vi "读取数据解析(子VI).vi"(6 "数据":string, 7 "命令编码CN":string, 11 "队列输入":refnum<queue>) -> (0 "实时数据发送时间间隔/min":i32=1, 1 "元素":T1(ring), 2 "设置超时时间/min":i32=1, 3 "队列输出":refnum<queue>, 4 "table":string="提取监测仪表时间")   [LabVIEW 2016, in "数据传输系统.lvlib"]
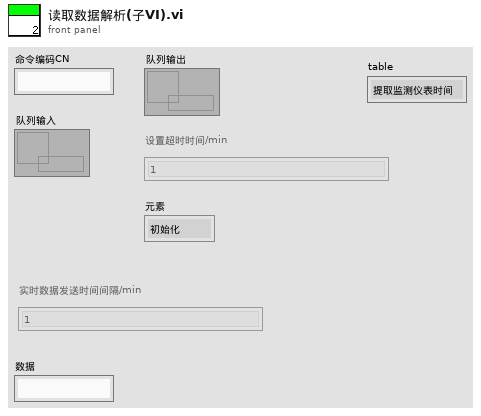
[diagram p1: front panel]
types:
  T1 = enum16{"初始化", "打开连接", "表格比对", "发送数据", "读取数据", "数据处理"}
  T2 = enum16{"CODMn", "CODCr", "氨氮", "总磷", "总氮", "数采仪"}
  T3 = cluster{"高锰酸盐":string, "化学需氧量":string, "氨氮":string, "总磷":string, "总氮":string, "数采仪":string, "高锰酸盐":bool, "化学需氧量":bool, "氨氮":bool, "总磷":bool, "总氮":bool, "数采仪":bool}
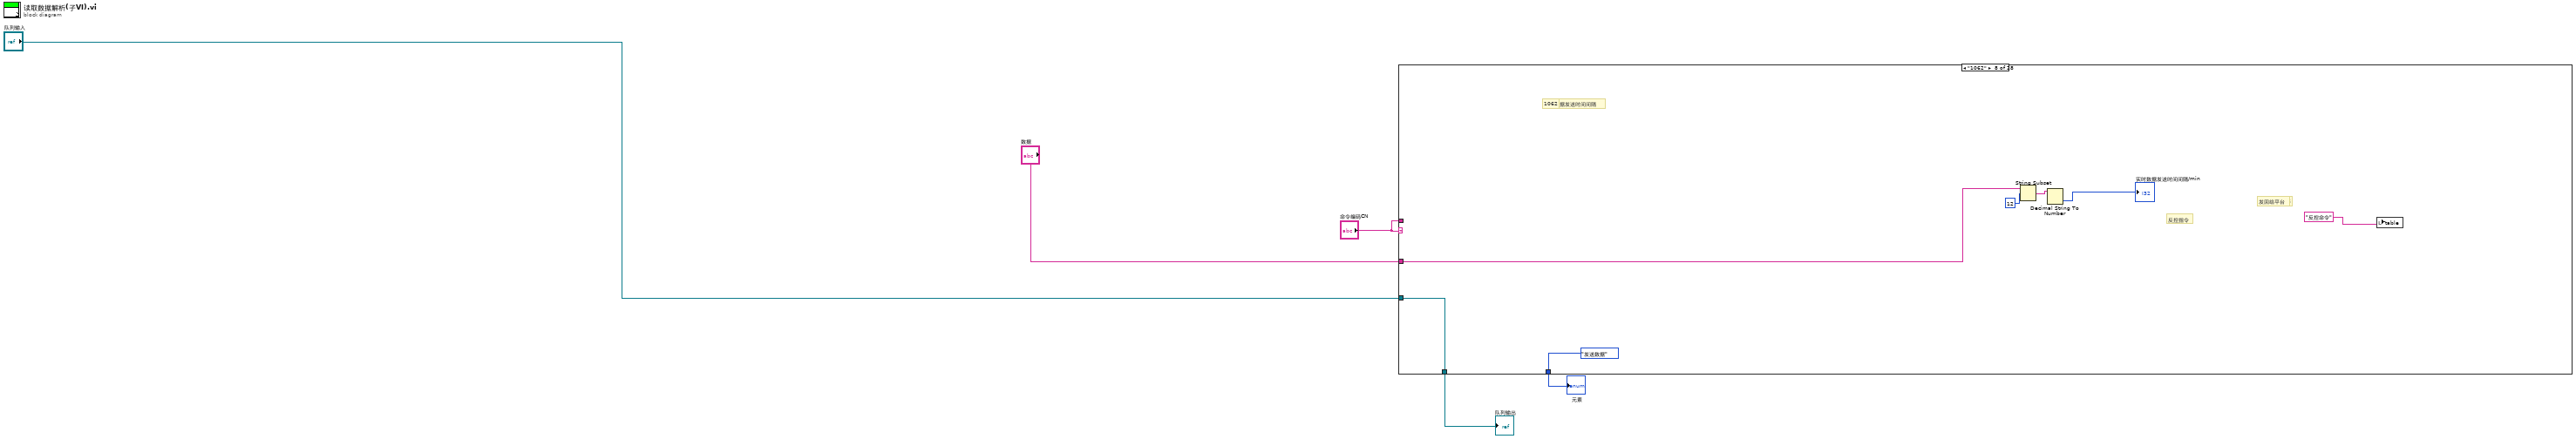
[diagram p0: block diagram]
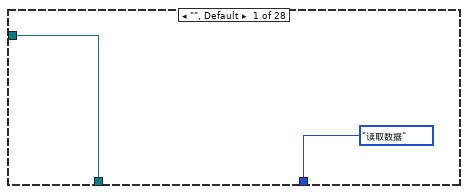
[diagram p2: hidden frame]
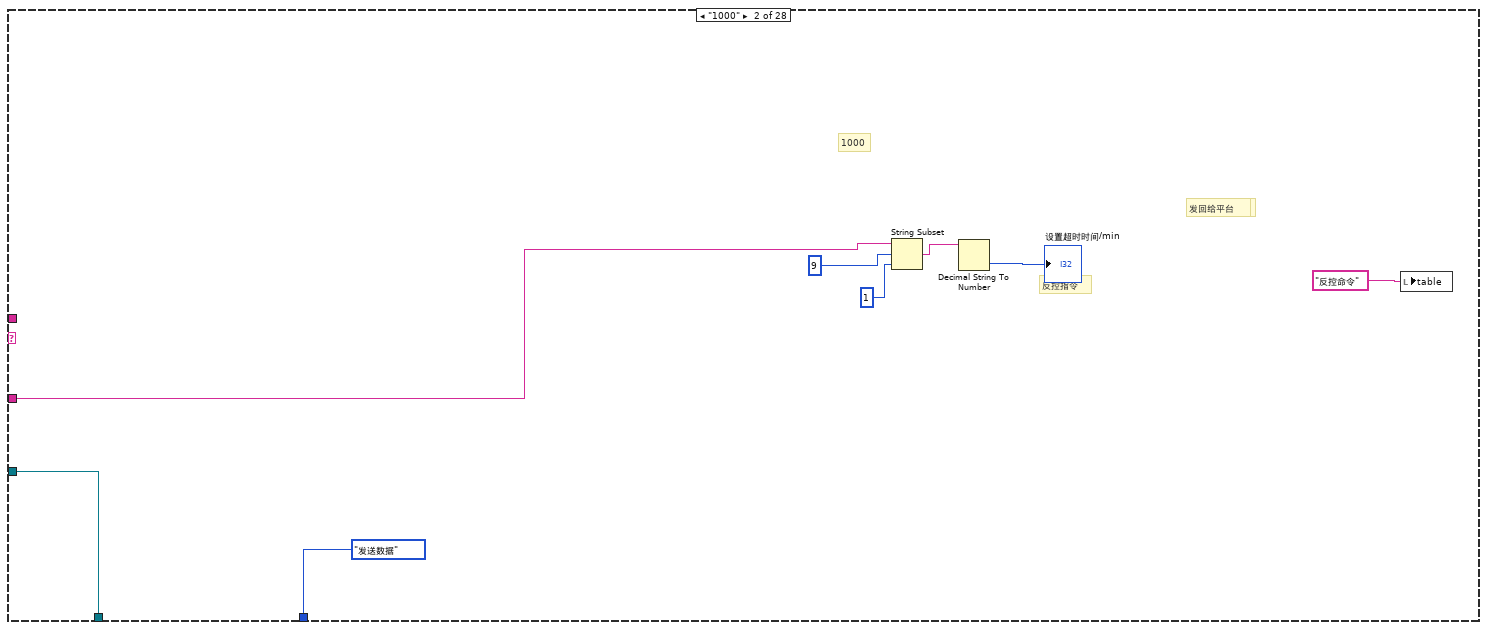
[diagram p3: hidden frame]
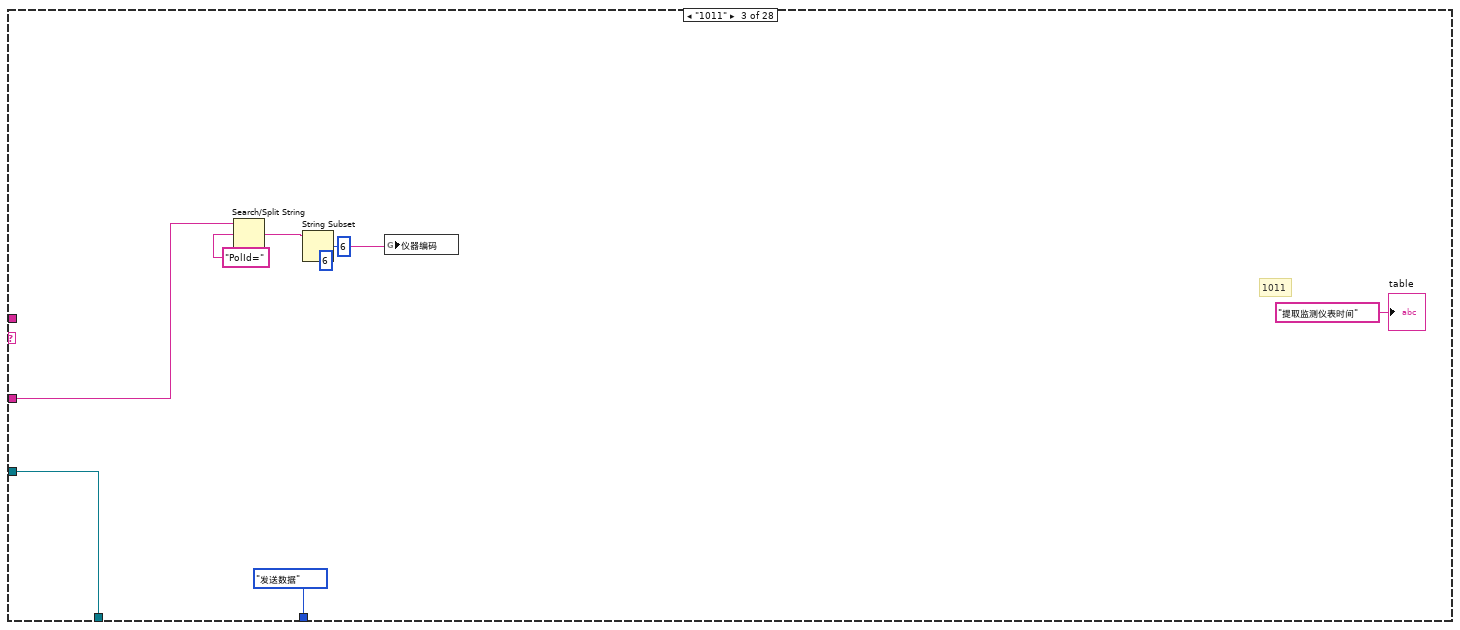
[diagram p4: hidden frame]
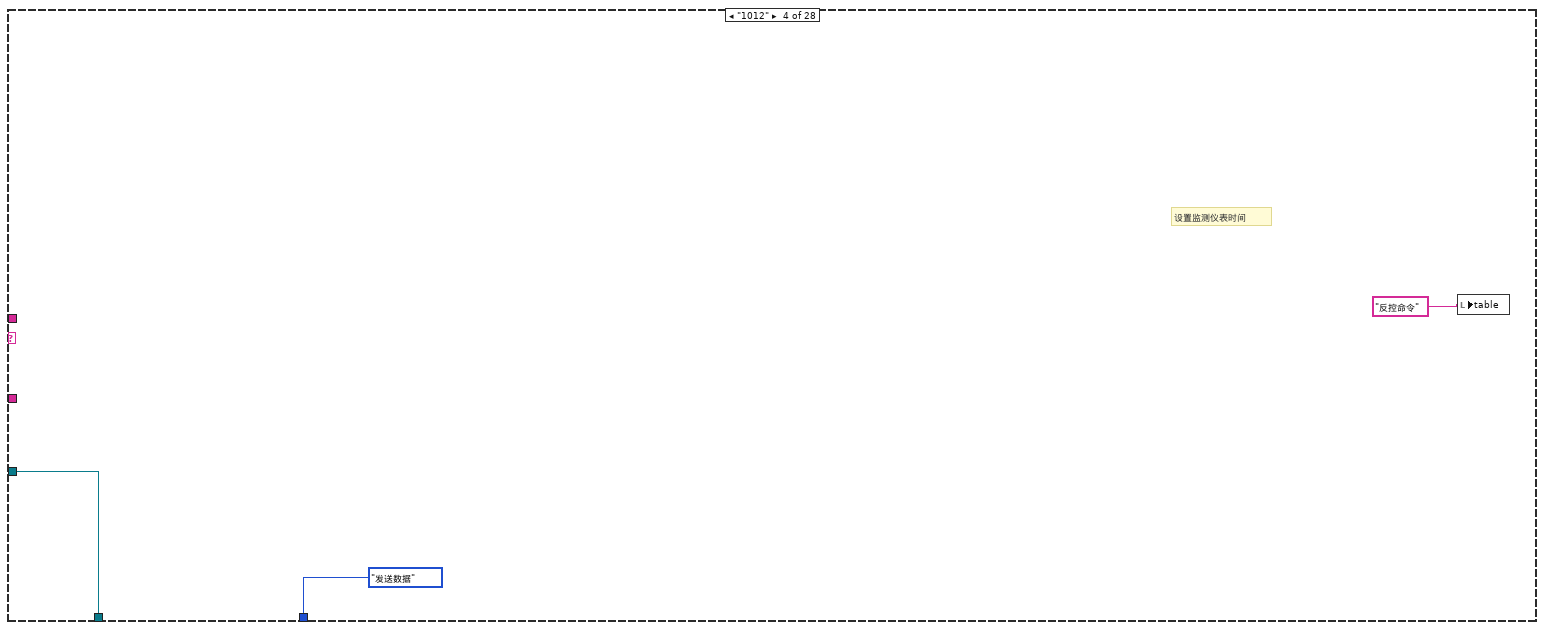
[diagram p5: hidden frame]
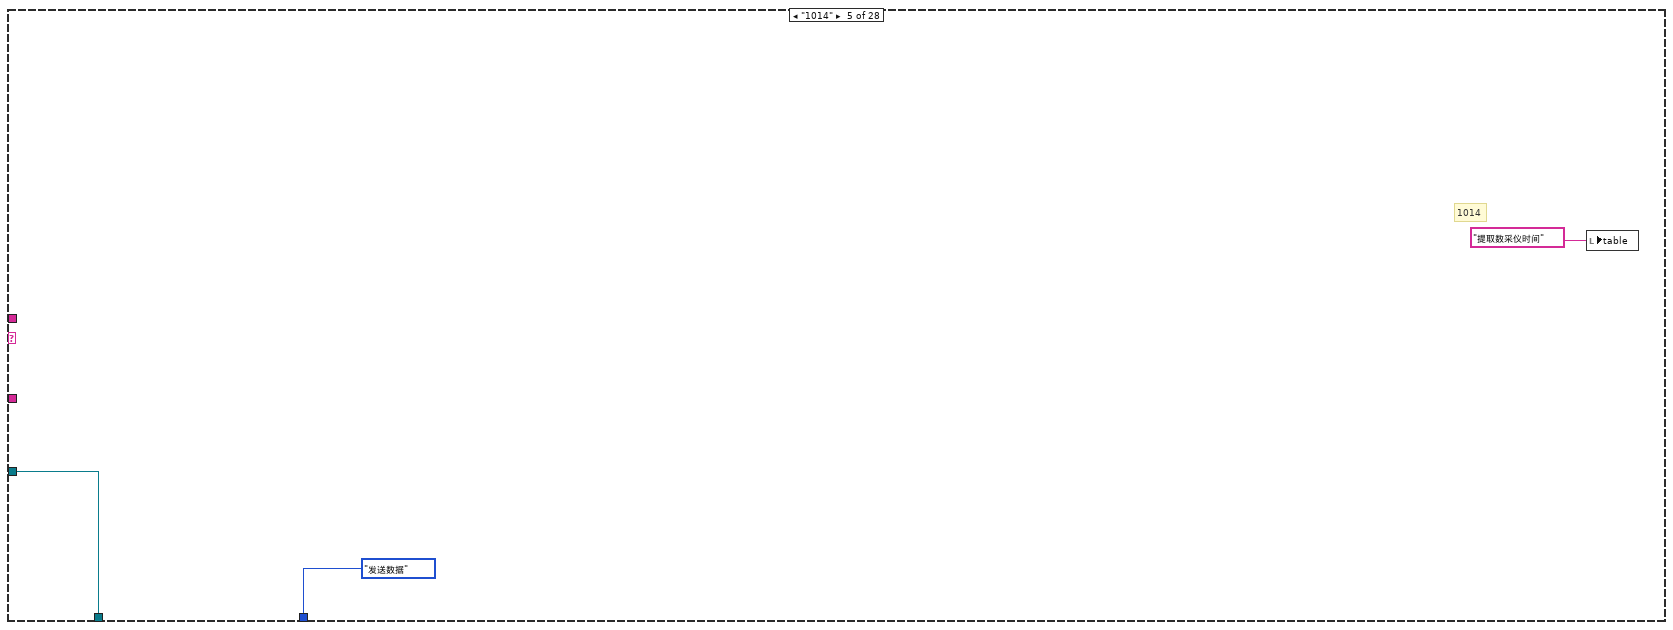
[diagram p6: hidden frame]
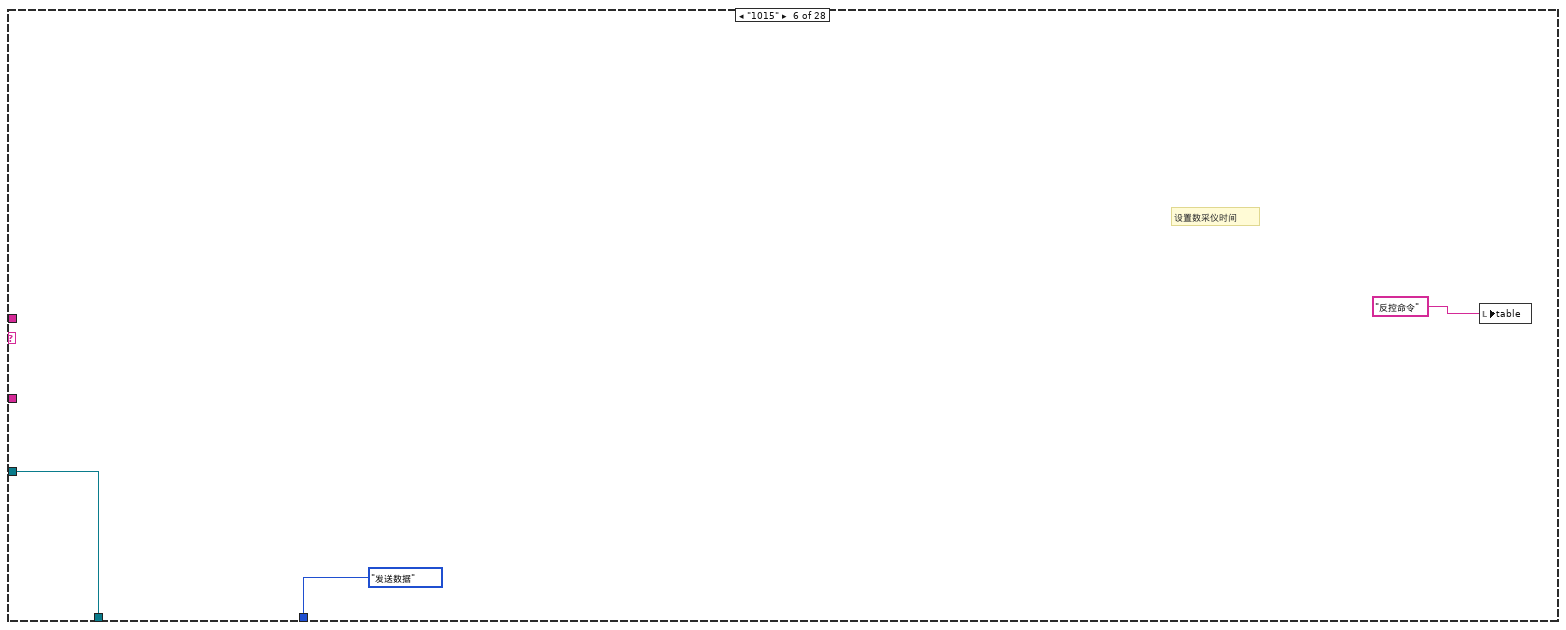
[diagram p7: hidden frame]
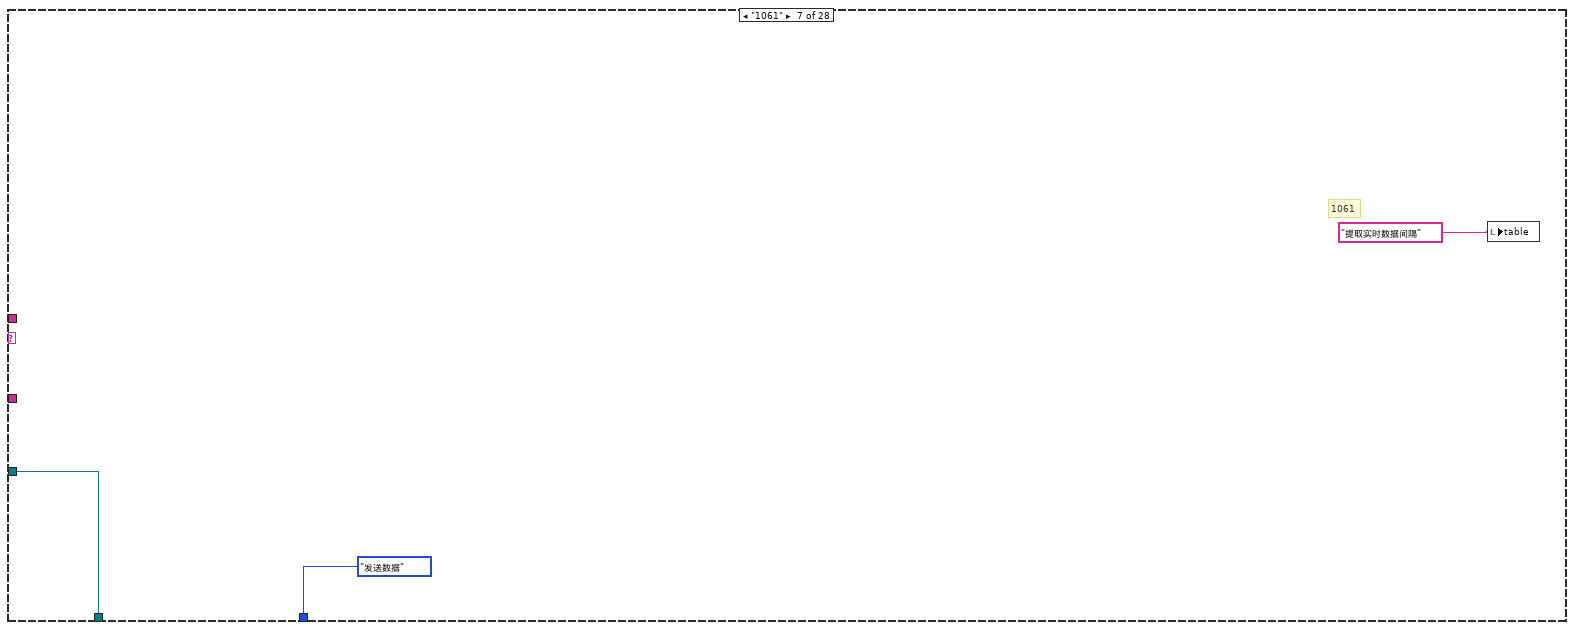
[diagram p8: hidden frame]
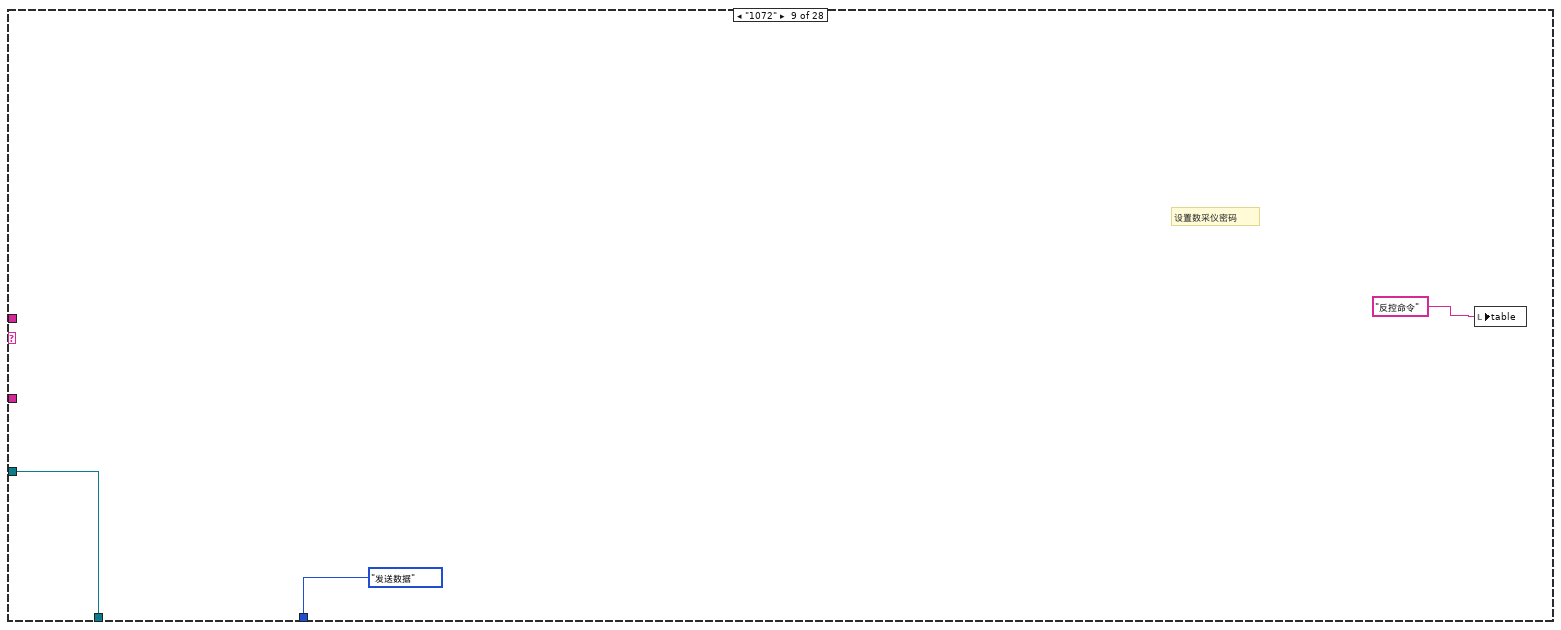
[diagram p9: hidden frame]
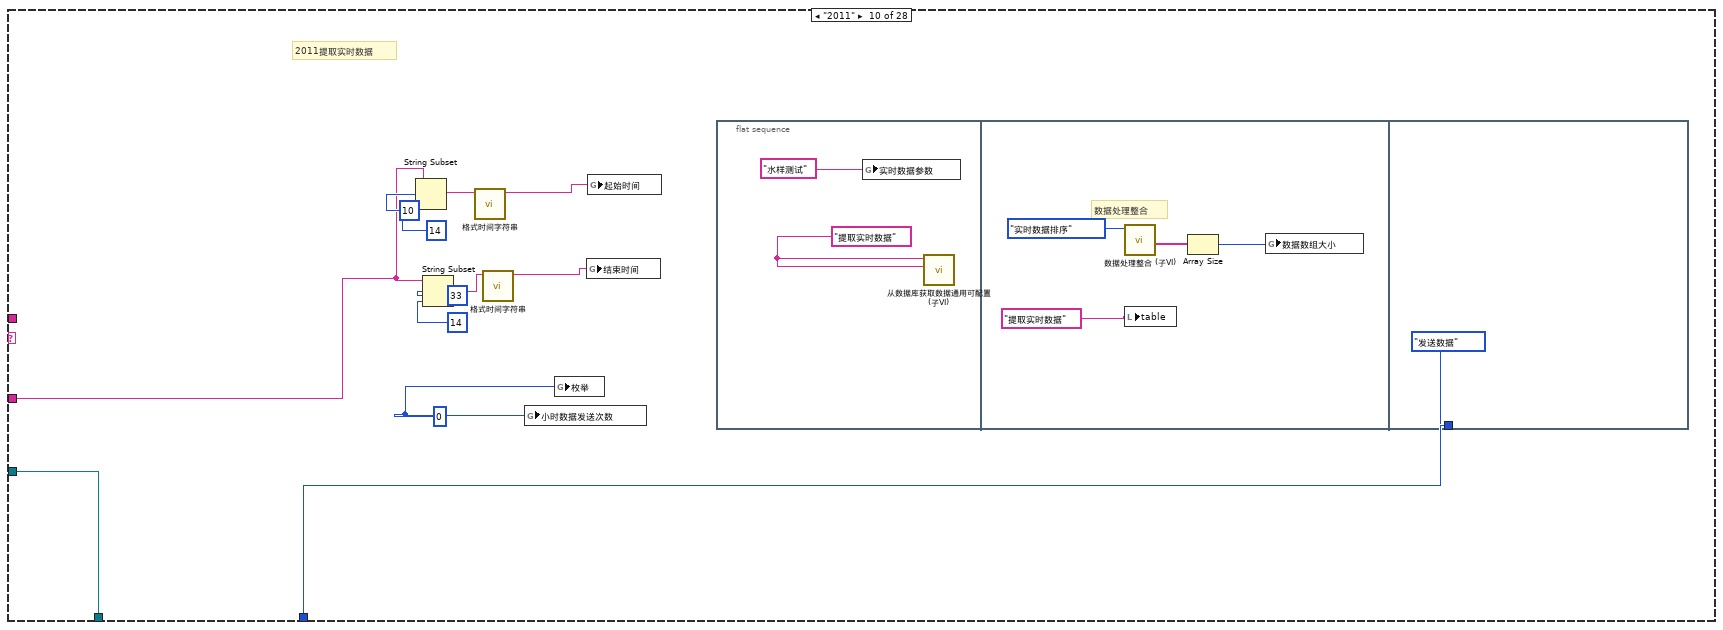
[diagram p10: hidden frame]
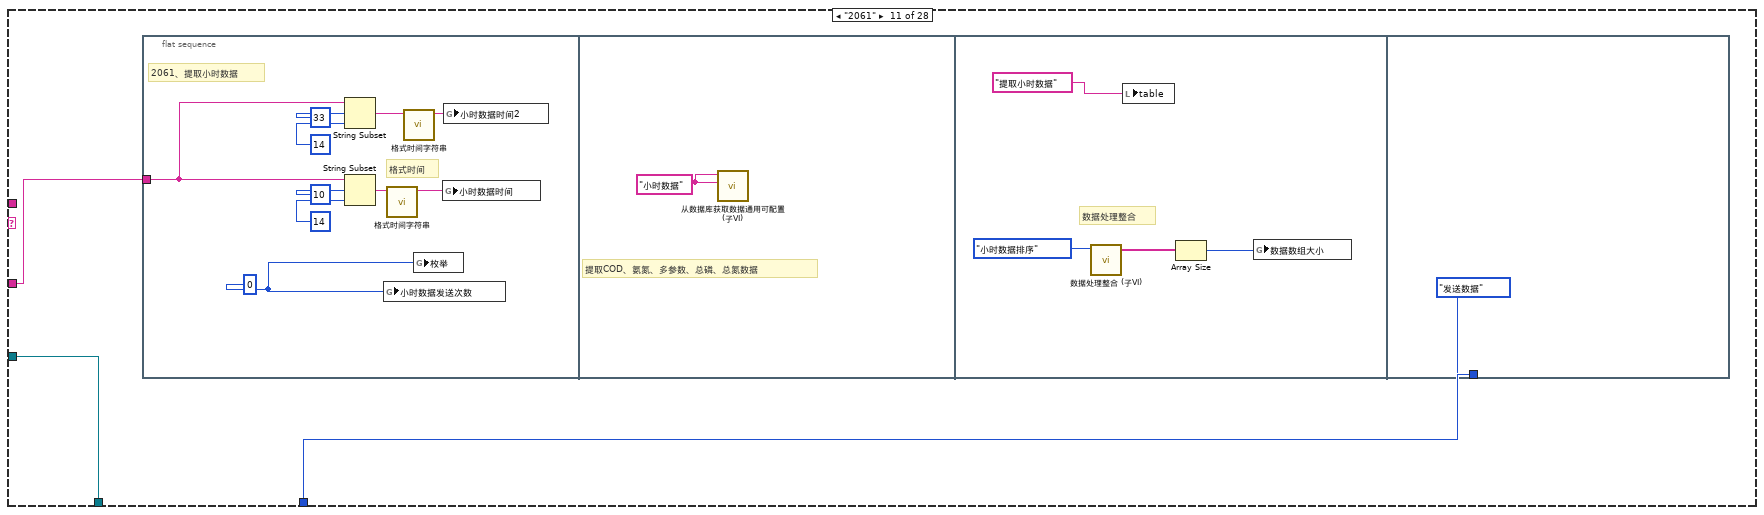
[diagram p11: hidden frame]
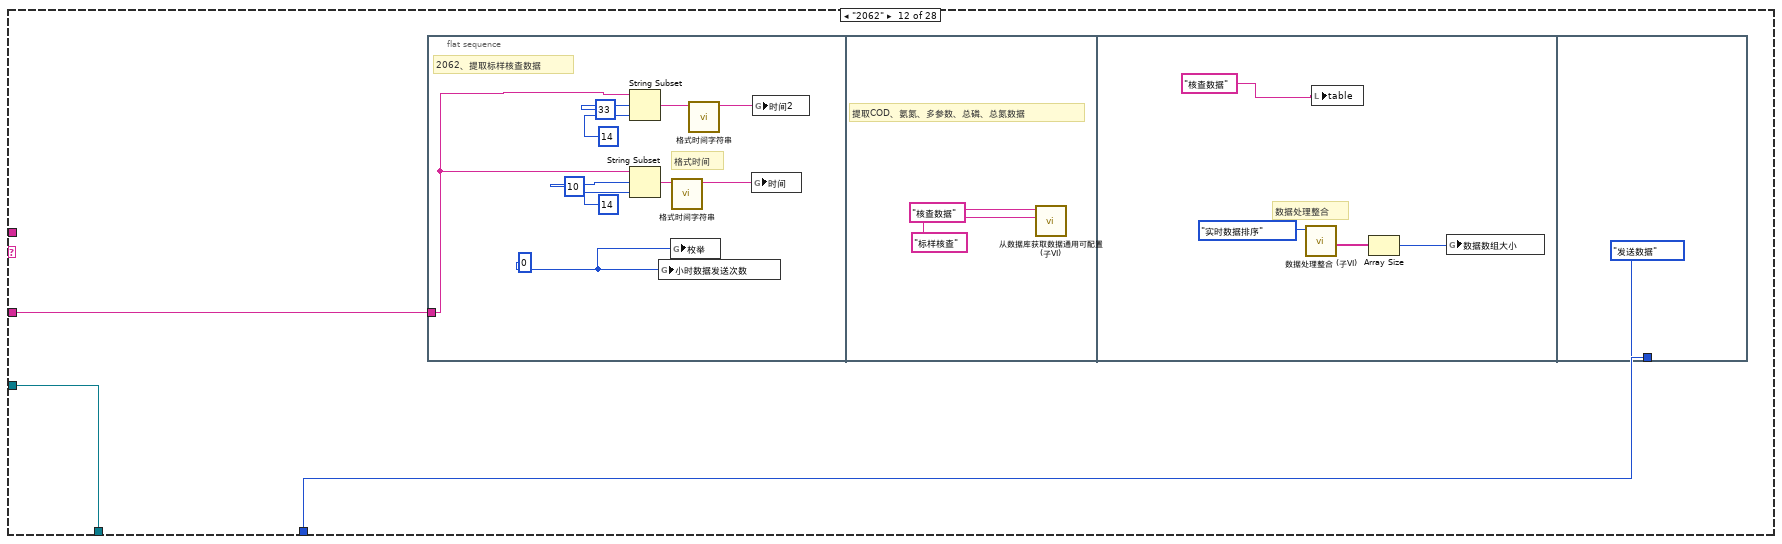
[diagram p12: hidden frame]
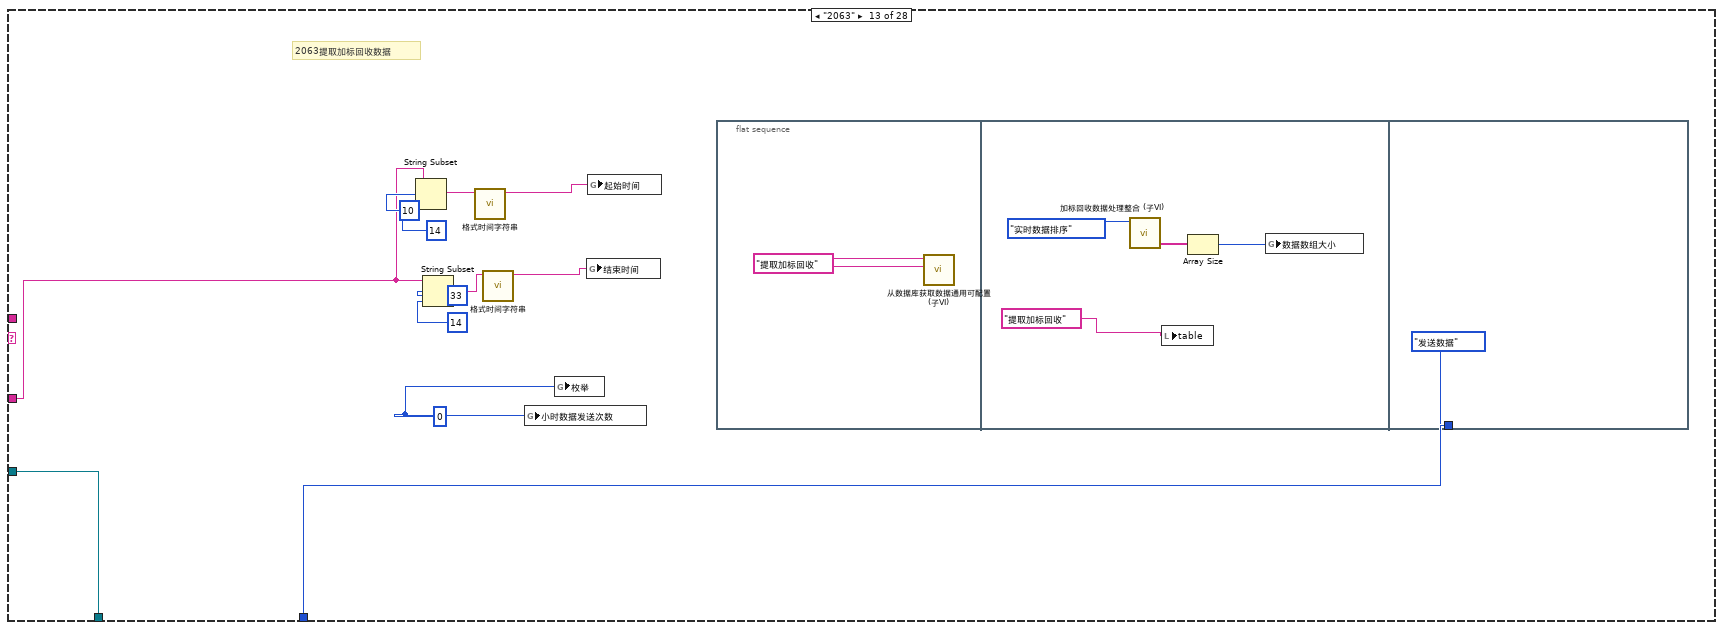
[diagram p13: hidden frame]
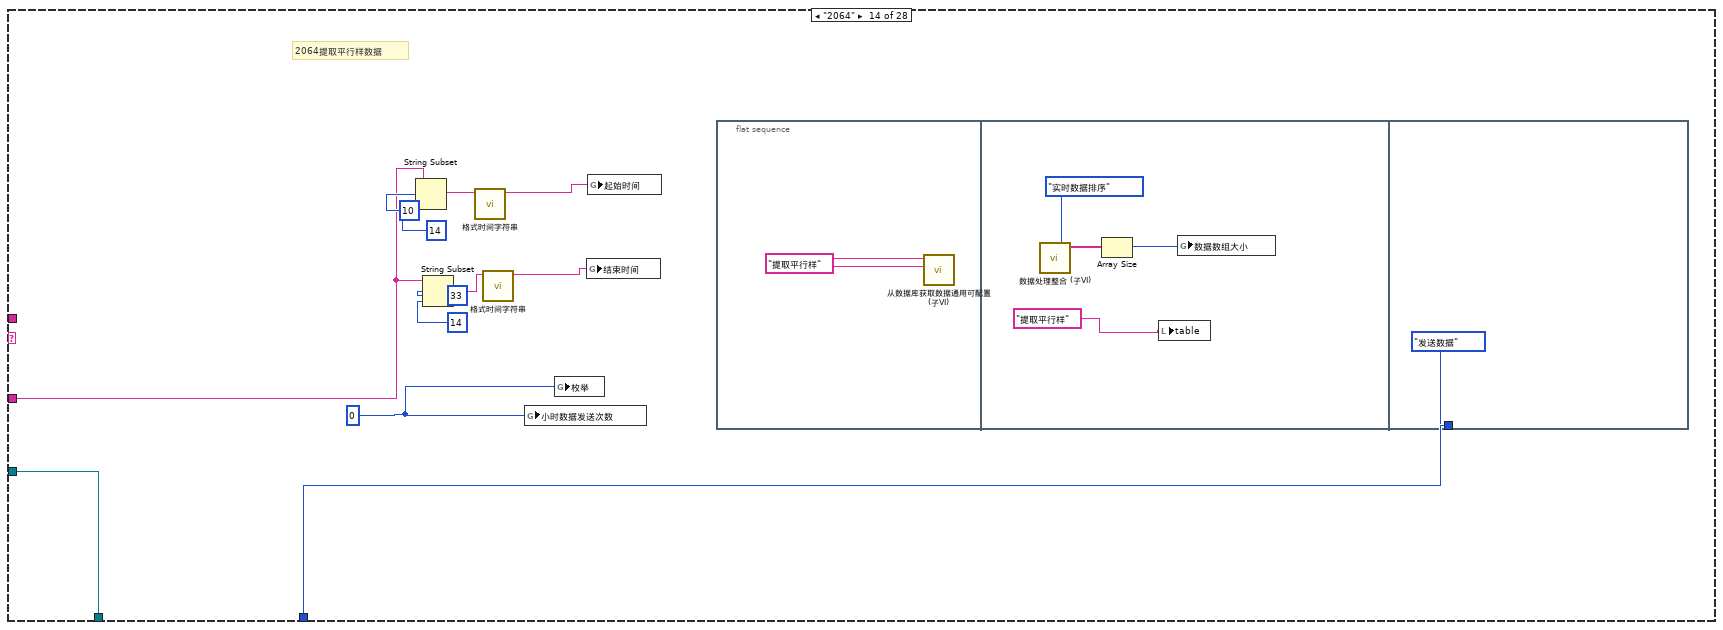
[diagram p14: hidden frame]
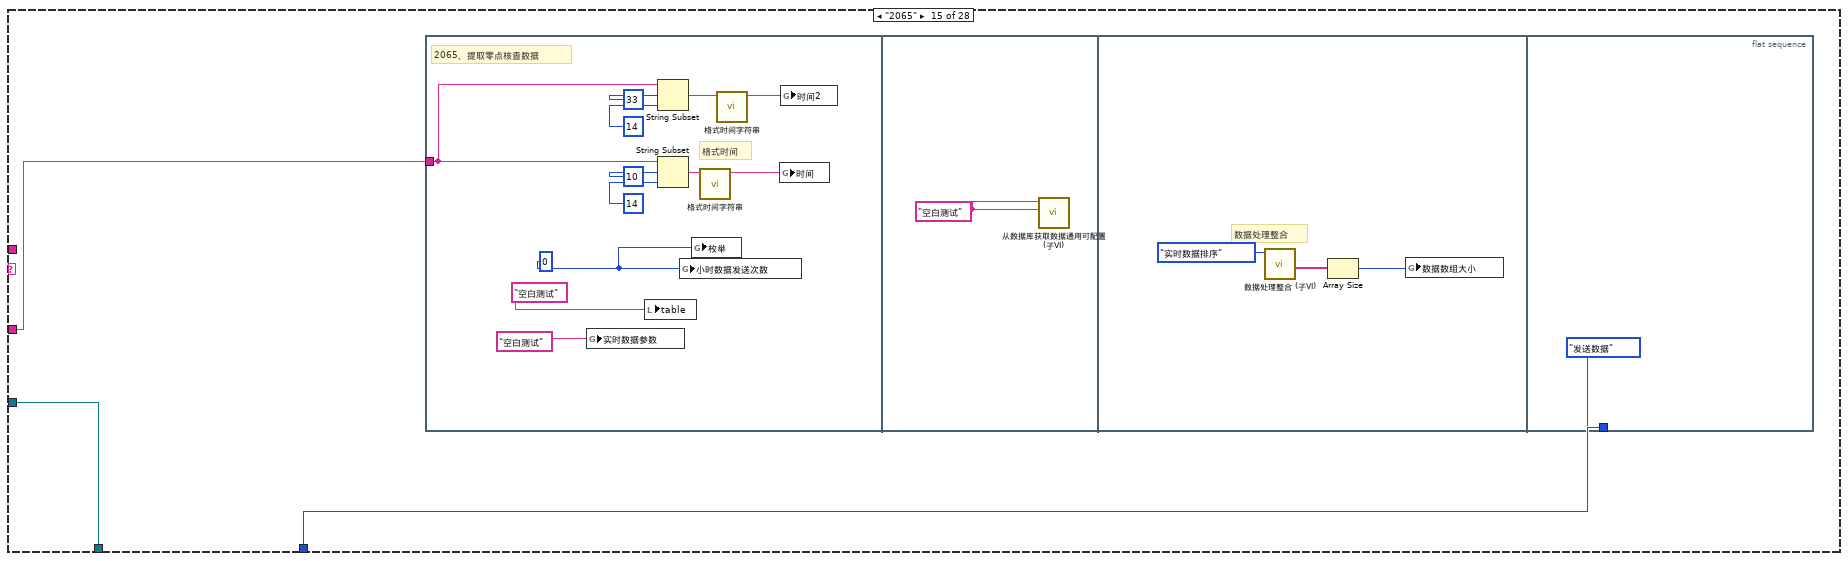
[diagram p15: hidden frame]
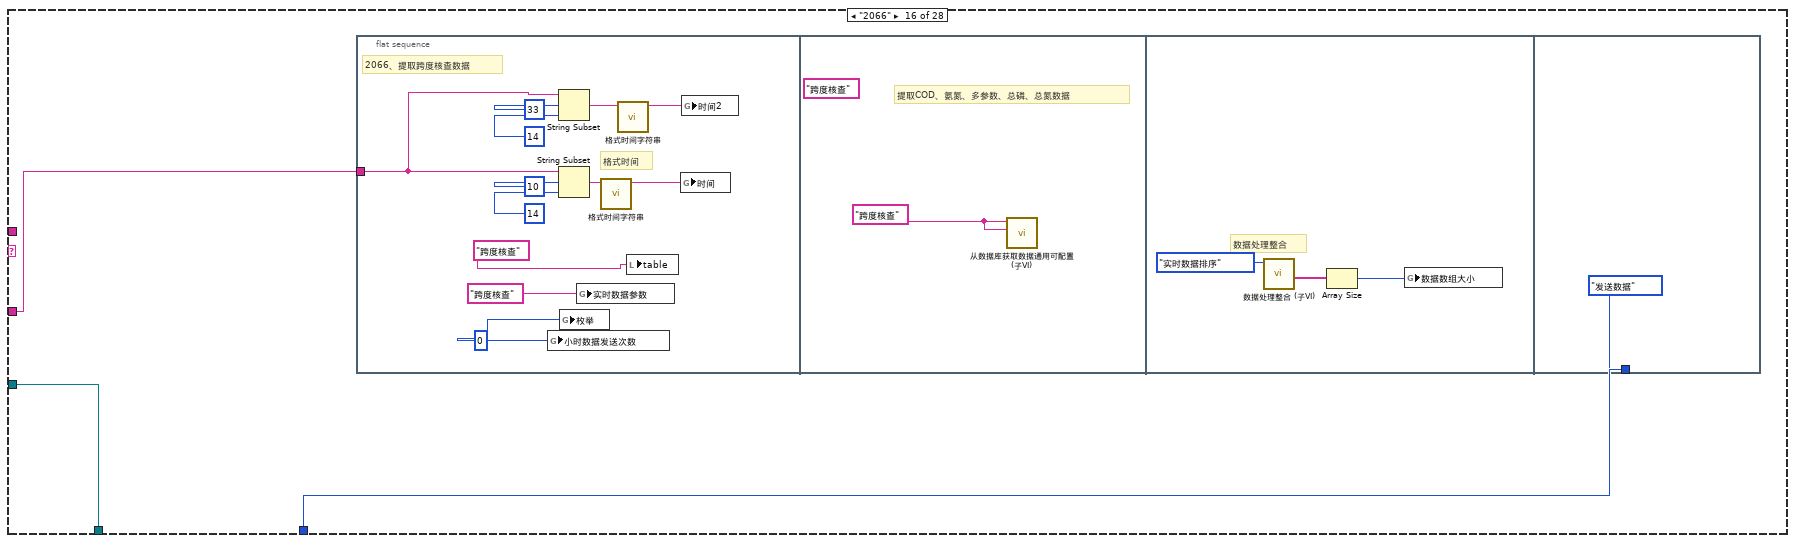
[diagram p16: hidden frame]
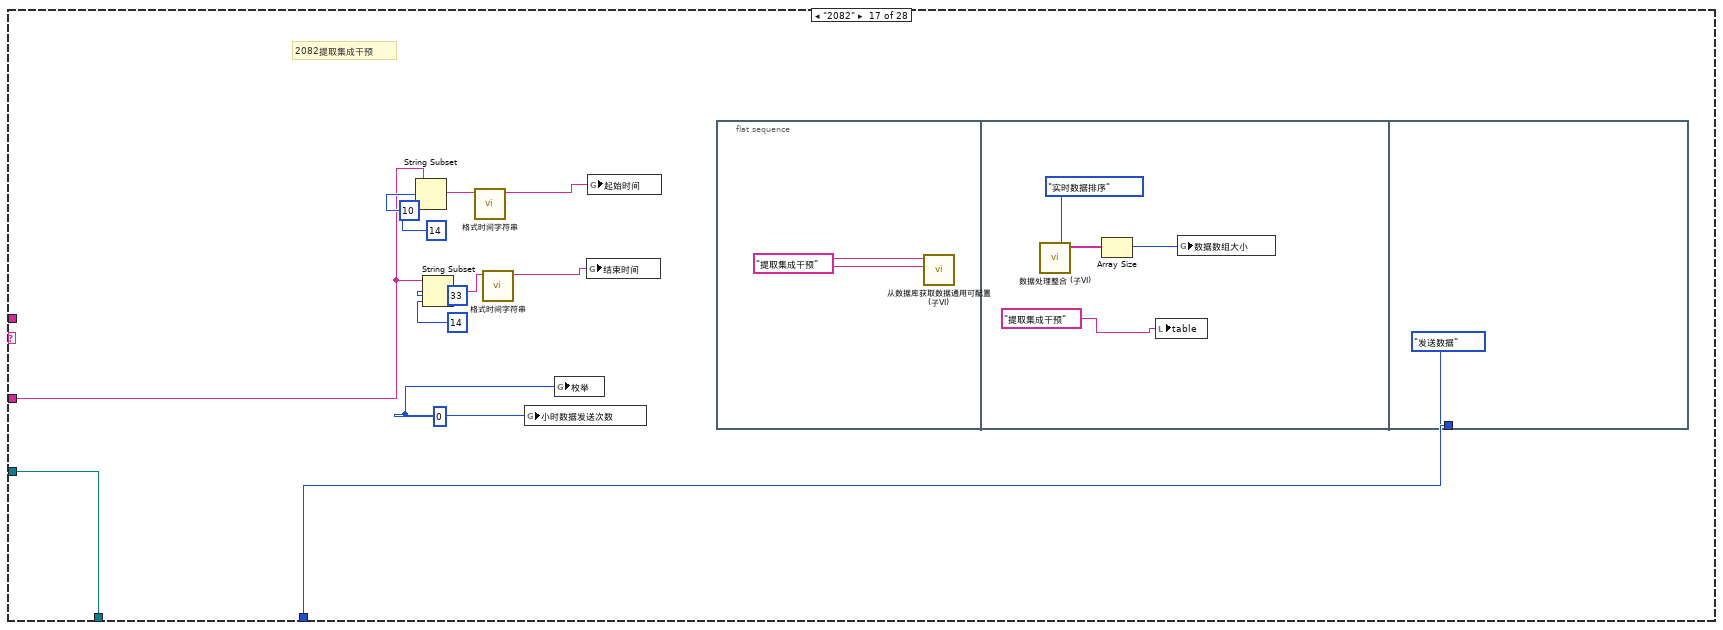
[diagram p17: hidden frame]
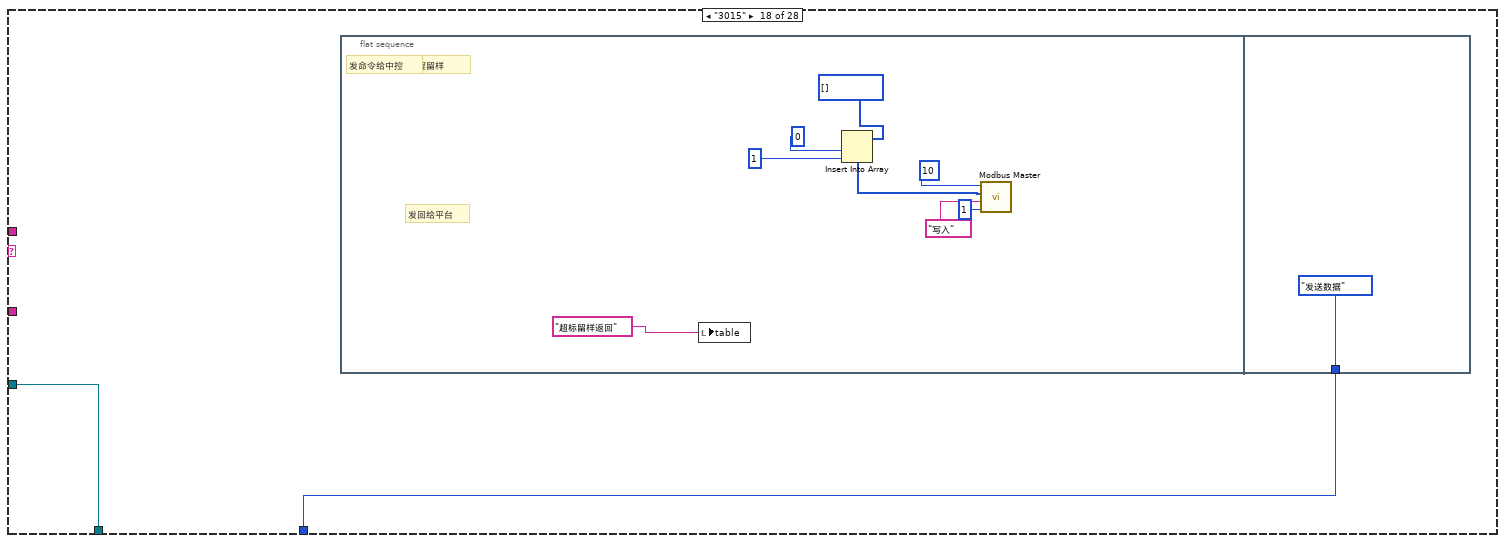
[diagram p18: hidden frame]
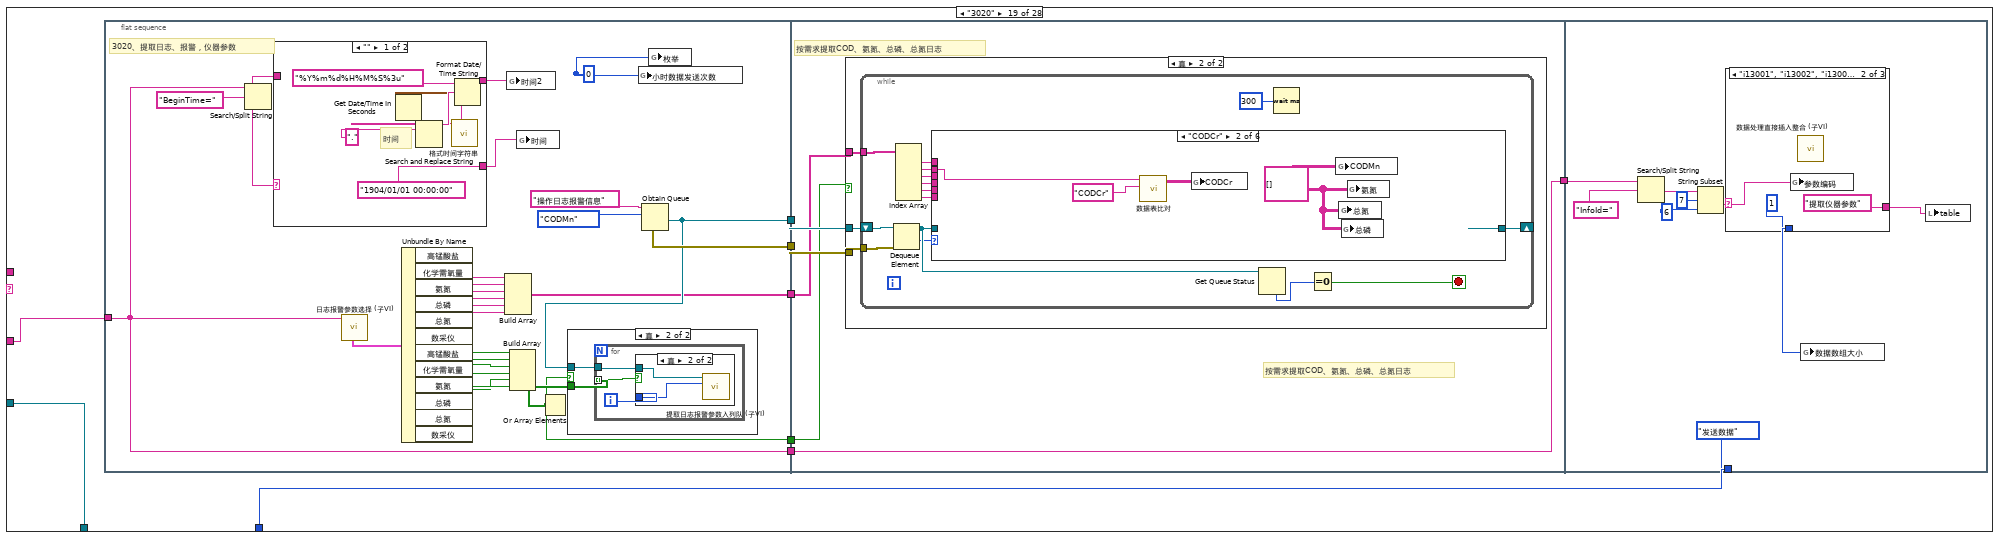
[diagram p19: hidden frame]
diagram:
  n1 = case shown="\"1062\"" "命令编码CN" {
    tunnel: "队列输入" -> [w7 w11 w24 w27 w30 w33 w36 w41 w46 w49 w68 w87 w107 w125 w143 w163 w183 w200 w218 w341 w343 w347 w355 w372 w375 w387 w409 w416]
    tunnel: [w7 w11 w24 w27 w30 w33 w36 w41 w46 w49 w68 w87 w107 w125 w143 w163 w183 w200 w218 w341 w343 w347 w355 w372 w375 w387 w409 w416] -> w2
    tunnel: [T1."读取数据" ("元素") T1."发送数据" ("元素") T1."发送数据" ("元素") T1."发送数据" ("元素") T1."发送数据" ("元素") T1."发送数据" ("元素") T1."发送数据" ("元素") T1."发送数据" ("元素") T1."发送数据" ("元素") w48 w67 w86 w106 w124 w142 w162 w182 w199 w217 T1."发送数据" ("元素") w342 w346 T1."发送数据" ("元素") T1."发送数据" ("元素") T1."发送数据" ("元素") T1."发送数据" ("元素") T1."发送数据" ("元素") T1."发送数据" ("元素")] -> w3
    tunnel: "命令编码CN" -> [_ _ _ _ _ _ _ _ _ _ _ _ _ _ _ _ _ _ _ _ _ _ _ _ _ _ _ w415]
    tunnel: "数据" -> [_ w9 w17 _ _ _ _ w39 _ w47 w66 w85 w105 w123 w141 w161 w181 _ w212 _ _ _ w351 _ _ _ w398 w412]
    frame "", Default {
    }
    frame "1000" {
      # "发回给平台"
      # "反控指令"
      # "3042~3086"
      # "1000"
      n2 = String Subset(string=w9, offset (0)=9 ("偏移量(0)"), length (rest)=1 ("长度（剩余）")) -> (substring=w13:string)
      n3 = Decimal String To Number(string=w13) -> (number=→"设置超时时间/min":i32)  [unwired: 2 in, 1 out]
      n4 = local write "table"("反控命令" ("新元素/子数组")) -> ()
    }
    frame "1011" {
      # "1011"
      n5 = Search/Split String(string=w17, search string/char (-)="PolId=" ("搜索字符串/字符(-)")) -> (match + rest of string=w21:string)  [unwired: 1 in, 2 out]
      n6 = String Subset(string=w21, offset (0)=6 ("偏移量(0)"), length (rest)=6 ("长度（剩余）")) -> (substring=w18:string)
      n7 = global write "全局 提取仪器参数.vi" "仪器编码"(w18) -> ()
      "table" <- "提取监测仪表时间"
    }
    frame "1012" {
      # "设置监测仪表时间"
      n8 = local write "table"("反控命令" ("新元素/子数组")) -> ()
    }
    frame "1014" {
      # "1014"
      n9 = local write "table"("提取数采仪时间") -> ()
    }
    frame "1015" {
      # "设置数采仪时间"
      n10 = local write "table"("反控命令" ("新元素/子数组")) -> ()
    }
    frame "1061" {
      # "1061"
      n11 = local write "table"("提取实时数据间隔") -> ()
    }
    frame "1062" {
      # "发回给平台"
      # "反控指令"
      # "3042~3086"
      # "设置数据发送时间间隔"
      # "1062"
      n12 = String Subset(string=w39, offset (0)=12 ("偏移量(0)")) -> (substring=w42:string)  [unwired: 1 in]
      n13 = Decimal String To Number(string=w42) -> (number=→"实时数据发送时间间隔/min":i32)  [unwired: 2 in, 1 out]
      n14 = local write "table"("反控命令" ("新元素/子数组")) -> ()
    }
    frame "1072" {
      # "设置数采仪密码"
      n15 = local write "table"("反控命令" ("新元素/子数组")) -> ()
    }
    frame "2011" {
      w54 = 0 ("数值")
      # "2011提取实时数据"
      n16 = String Subset(string=w47, offset (0)=10 ("偏移量(0)"), length (rest)=14 ("长度（剩余）")) -> (substring=w51:string)
      n17 = String Subset(string=w47, offset (0)=33 ("偏移量(0)"), length (rest)=14 ("长度（剩余）")) -> (substring=w53:string)
      n18 = call "格式时间字符串.vi"("字符串"=w51) -> ("连接的字符串"=w50:string)  [unwired: 10 in]
      n19 = call "格式时间字符串.vi"("字符串"=w53) -> ("连接的字符串"=w52:string)  [unwired: 10 in]
      n20 = global write "全局 小时数据发送次数.vi" "小时数据发送次数"(w54) -> ()
      n21 = global write "全局1.vi" "枚举"(w54) -> ()
      n22 = global write "起始时间.vi" "结束时间"(w52) -> ()
      n23 = global write "起始时间.vi" "起始时间"(w50) -> ()
      n24 = flat-sequence {
        tunnel: [T1."发送数据" ("元素")] -> w48
        frame #0 {
          w59 = "提取实时数据" ("新元素/子数组")
          n25 = global write "全局 实时数据参数.vi" "实时数据参数"("水样测试") -> ()
          n26 = call "从数据库获取数据通用可配置(子VI).vi"("table输入"=w59, "列队名（唯一）"=w59) -> ()  [unwired: 8 in, 2 out]
        }
        frame #1 {
          # "数据处理整合"
          n27 = call "数据处理整合 (子VI).vi"("枚举"=enum16{"实时数据排序", "小时数据排序"}."实时数据排序") -> ("已排序的数组"=w63:string[])  [unwired: 10 in]
          n28 = local write "table"("提取实时数据" ("新元素/子数组")) -> ()
          n29 = Array Size(array=w63) -> (size(s)=w64:i32)
          n30 = global write "全局 数据数组大小.vi" "数据数组大小"(w64) -> ()
        }
        frame #2 {
        }
      }
    }
    frame "2061" {
      n31 = flat-sequence {
        tunnel: w66 -> [w69]
        tunnel: [T1."发送数据" ("元素")] -> w67
        frame #0 {
          w70 = 0 ("数值")
          # "格式时间"
          # "2061、提取小时数据"
          n32 = String Subset(string=w69, offset (0)=33 ("偏移量(0)"), length (rest)=14 ("长度（剩余）")) -> (substring=w72:string)
          n33 = String Subset(string=w69, offset (0)=10 ("偏移量(0)"), length (rest)=14 ("长度（剩余）")) -> (substring=w73:string)
          n34 = global write "全局 小时数据发送次数.vi" "小时数据发送次数"(w70) -> ()
          n35 = call "格式时间字符串.vi"("字符串"=w73) -> ("连接的字符串"=w74:string)  [unwired: 10 in]
          n36 = call "格式时间字符串.vi"("字符串"=w72) -> ("连接的字符串"=w71:string)  [unwired: 10 in]
          n37 = global write "全局1.vi" "枚举"(w70) -> ()
          n38 = global write "全局 水样时间.vi" "小时数据时间"(w74) -> ()
          n39 = global write "全局 时间2.vi" "小时数据时间2"(w71) -> ()
        }
        frame #1 {
          w79 = "小时数据" ("名称（未命名）")
          # "提取COD、氨氮、多参数、总磷、总氮数据"
          n40 = call "从数据库获取数据通用可配置(子VI).vi"("table输入"=w79, "列队名（唯一）"=w79) -> ()  [unwired: 8 in, 2 out]
        }
        frame #2 {
          # "数据处理整合"
          n41 = call "数据处理整合 (子VI).vi"("枚举"=enum16{"实时数据排序", "小时数据排序"}."小时数据排序") -> ("已排序的数组"=w83:string[])  [unwired: 10 in]
          n42 = local write "table"("提取小时数据" ("新元素/子数组")) -> ()
          n43 = Array Size(array=w83) -> (size(s)=w82:i32)
          n44 = global write "全局 数据数组大小.vi" "数据数组大小"(w82) -> ()
        }
        frame #3 {
        }
      }
    }
    frame "2062" {
      n45 = flat-sequence {
        tunnel: w85 -> [w88]
        tunnel: [T1."发送数据" ("元素")] -> w86
        frame #0 {
          w89 = 0 ("数值")
          # "格式时间"
          # "2062、提取标样核查数据"
          n46 = String Subset(string=w88, offset (0)=33 ("偏移量(0)"), length (rest)=14 ("长度（剩余）")) -> (substring=w91:string)
          n47 = String Subset(string=w88, offset (0)=10 ("偏移量(0)"), length (rest)=14 ("长度（剩余）")) -> (substring=w92:string)
          n48 = global write "全局 小时数据发送次数.vi" "小时数据发送次数"(w89) -> ()
          n49 = global write "全局1.vi" "枚举"(w89) -> ()
          n50 = call "格式时间字符串.vi"("字符串"=w92) -> ("连接的字符串"=w93:string)  [unwired: 10 in]
          n51 = call "格式时间字符串.vi"("字符串"=w91) -> ("连接的字符串"=w90:string)  [unwired: 10 in]
          n52 = global write "全局 水样时间.vi" "时间"(w93) -> ()
          n53 = global write "全局 时间2.vi" "时间2"(w90) -> ()
        }
        frame #1 {
          # "提取COD、氨氮、多参数、总磷、总氮数据"
          n54 = call "从数据库获取数据通用可配置(子VI).vi"("table输入"="标样核查" ("新元素/子数组"), "列队名（唯一）"="核查数据" ("新元素/子数组")) -> ()  [unwired: 8 in, 2 out]
        }
        frame #2 {
          # "数据处理整合"
          n55 = call "数据处理整合 (子VI).vi"("枚举"=enum16{"实时数据排序", "小时数据排序"}."实时数据排序") -> ("已排序的数组"=w102:string[])  [unwired: 10 in]
          n56 = local write "table"("核查数据" ("新元素/子数组")) -> ()
          n57 = Array Size(array=w102) -> (size(s)=w103:i32)
          n58 = global write "全局 数据数组大小.vi" "数据数组大小"(w103) -> ()
        }
        frame #3 {
        }
      }
    }
    frame "2063" {
      w112 = 0 ("数值")
      # "2063提取加标回收数据"
      n59 = String Subset(string=w105, offset (0)=10 ("偏移量(0)"), length (rest)=14 ("长度（剩余）")) -> (substring=w109:string)
      n60 = String Subset(string=w105, offset (0)=33 ("偏移量(0)"), length (rest)=14 ("长度（剩余）")) -> (substring=w111:string)
      n61 = call "格式时间字符串.vi"("字符串"=w109) -> ("连接的字符串"=w108:string)  [unwired: 10 in]
      n62 = call "格式时间字符串.vi"("字符串"=w111) -> ("连接的字符串"=w110:string)  [unwired: 10 in]
      n63 = global write "全局 小时数据发送次数.vi" "小时数据发送次数"(w112) -> ()
      n64 = global write "全局1.vi" "枚举"(w112) -> ()
      n65 = global write "起始时间.vi" "结束时间"(w110) -> ()
      n66 = global write "起始时间.vi" "起始时间"(w108) -> ()
      n67 = flat-sequence {
        tunnel: [T1."发送数据" ("元素")] -> w106
        frame #0 {
          w117 = "提取加标回收" ("新元素/子数组")
          n68 = call "从数据库获取数据通用可配置(子VI).vi"("table输入"=w117, "列队名（唯一）"=w117) -> ()  [unwired: 8 in, 2 out]
        }
        frame #1 {
          n69 = call "加标回收数据处理整合 (子VI).vi"("枚举"=enum16{"实时数据排序", "小时数据排序"}."实时数据排序") -> ("已排序的数组"=w119:string[])  [unwired: 10 in]
          n70 = local write "table"("提取加标回收" ("新元素/子数组")) -> ()
          n71 = Array Size(array=w119) -> (size(s)=w121:i32)
          n72 = global write "全局 数据数组大小.vi" "数据数组大小"(w121) -> ()
        }
        frame #2 {
        }
      }
    }
    frame "2064" {
      w130 = 0 ("数值")
      # "2064提取平行样数据"
      n73 = String Subset(string=w123, offset (0)=10 ("偏移量(0)"), length (rest)=14 ("长度（剩余）")) -> (substring=w127:string)
      n74 = String Subset(string=w123, offset (0)=33 ("偏移量(0)"), length (rest)=14 ("长度（剩余）")) -> (substring=w129:string)
      n75 = call "格式时间字符串.vi"("字符串"=w127) -> ("连接的字符串"=w126:string)  [unwired: 10 in]
      n76 = call "格式时间字符串.vi"("字符串"=w129) -> ("连接的字符串"=w128:string)  [unwired: 10 in]
      n77 = global write "全局 小时数据发送次数.vi" "小时数据发送次数"(w130) -> ()
      n78 = global write "全局1.vi" "枚举"(w130) -> ()
      n79 = global write "起始时间.vi" "结束时间"(w128) -> ()
      n80 = global write "起始时间.vi" "起始时间"(w126) -> ()
      n81 = flat-sequence {
        tunnel: [T1."发送数据" ("元素")] -> w124
        frame #0 {
          w135 = "提取平行样" ("新元素/子数组")
          n82 = call "从数据库获取数据通用可配置(子VI).vi"("table输入"=w135, "列队名（唯一）"=w135) -> ()  [unwired: 8 in, 2 out]
        }
        frame #1 {
          n83 = call "数据处理整合 (子VI).vi"("枚举"=enum16{"实时数据排序", "小时数据排序"}."实时数据排序") -> ("已排序的数组"=w139:string[])  [unwired: 10 in]
          n84 = Array Size(array=w139) -> (size(s)=w138:i32)
          n85 = local write "table"("提取平行样" ("新元素/子数组")) -> ()
          n86 = global write "全局 数据数组大小.vi" "数据数组大小"(w138) -> ()
        }
        frame #2 {
        }
      }
    }
    frame "2065" {
      n87 = flat-sequence {
        tunnel: w141 -> [w145]
        tunnel: [T1."发送数据" ("元素")] -> w142
        frame #0 {
          w146 = 0 ("数值")
          # "格式时间"
          # "2065、提取零点核查数据"
          n88 = global write "全局 实时数据参数.vi" "实时数据参数"("空白测试" ("新元素/子数组")) -> ()
          n89 = local write "table"("空白测试" ("新元素/子数组")) -> ()
          n90 = String Subset(string=w145, offset (0)=33 ("偏移量(0)"), length (rest)=14 ("长度（剩余）")) -> (substring=w149:string)
          n91 = String Subset(string=w145, offset (0)=10 ("偏移量(0)"), length (rest)=14 ("长度（剩余）")) -> (substring=w150:string)
          n92 = global write "全局 小时数据发送次数.vi" "小时数据发送次数"(w146) -> ()
          n93 = global write "全局1.vi" "枚举"(w146) -> ()
          n94 = call "格式时间字符串.vi"("字符串"=w150) -> ("连接的字符串"=w151:string)  [unwired: 10 in]
          n95 = call "格式时间字符串.vi"("字符串"=w149) -> ("连接的字符串"=w148:string)  [unwired: 10 in]
          n96 = global write "全局 水样时间.vi" "时间"(w151) -> ()
          n97 = global write "全局 时间2.vi" "时间2"(w148) -> ()
        }
        frame #1 {
          w156 = "空白测试" ("新元素/子数组")
          n98 = call "从数据库获取数据通用可配置(子VI).vi"("table输入"=w156, "列队名（唯一）"=w156) -> ()  [unwired: 8 in, 2 out]
        }
        frame #2 {
          # "数据处理整合"
          n99 = call "数据处理整合 (子VI).vi"("枚举"=enum16{"实时数据排序", "小时数据排序"}."实时数据排序") -> ("已排序的数组"=w158:string[])  [unwired: 10 in]
          n100 = Array Size(array=w158) -> (size(s)=w159:i32)
          n101 = global write "全局 数据数组大小.vi" "数据数组大小"(w159) -> ()
        }
        frame #3 {
        }
      }
    }
    frame "2066" {
      n102 = flat-sequence {
        tunnel: w161 -> [w165]
        tunnel: [T1."发送数据" ("元素")] -> w162
        frame #0 {
          w166 = 0 ("数值")
          # "格式时间"
          # "2066、提取跨度核查数据"
          n103 = global write "全局 小时数据发送次数.vi" "小时数据发送次数"(w166) -> ()
          n104 = String Subset(string=w165, offset (0)=33 ("偏移量(0)"), length (rest)=14 ("长度（剩余）")) -> (substring=w169:string)
          n105 = String Subset(string=w165, offset (0)=10 ("偏移量(0)"), length (rest)=14 ("长度（剩余）")) -> (substring=w170:string)
          n106 = global write "全局1.vi" "枚举"(w166) -> ()
          n107 = global write "全局 实时数据参数.vi" "实时数据参数"("跨度核查" ("新元素/子数组")) -> ()
          n108 = call "格式时间字符串.vi"("字符串"=w170) -> ("连接的字符串"=w171:string)  [unwired: 10 in]
          n109 = call "格式时间字符串.vi"("字符串"=w169) -> ("连接的字符串"=w168:string)  [unwired: 10 in]
          n110 = local write "table"("跨度核查" ("新元素/子数组")) -> ()
          n111 = global write "全局 水样时间.vi" "时间"(w171) -> ()
          n112 = global write "全局 时间2.vi" "时间2"(w168) -> ()
        }
        frame #1 {
          w176 = "跨度核查" ("新元素/子数组")
          (unwired) "跨度核查" ("名称（未命名）")
          # "提取COD、氨氮、多参数、总磷、总氮数据"
          n113 = call "从数据库获取数据通用可配置(子VI).vi"("table输入"=w176, "列队名（唯一）"=w176) -> ()  [unwired: 8 in, 2 out]
        }
        frame #2 {
          # "数据处理整合"
          n114 = call "数据处理整合 (子VI).vi"("枚举"=enum16{"实时数据排序", "小时数据排序"}."实时数据排序") -> ("已排序的数组"=w179:string[])  [unwired: 10 in]
          n115 = Array Size(array=w179) -> (size(s)=w178:i32)
          n116 = global write "全局 数据数组大小.vi" "数据数组大小"(w178) -> ()
        }
        frame #3 {
        }
      }
    }
    frame "2082" {
      w188 = 0 ("数值")
      # "2082提取集成干预"
      n117 = String Subset(string=w181, offset (0)=10 ("偏移量(0)"), length (rest)=14 ("长度（剩余）")) -> (substring=w185:string)
      n118 = String Subset(string=w181, offset (0)=33 ("偏移量(0)"), length (rest)=14 ("长度（剩余）")) -> (substring=w187:string)
      n119 = call "格式时间字符串.vi"("字符串"=w185) -> ("连接的字符串"=w184:string)  [unwired: 10 in]
      n120 = call "格式时间字符串.vi"("字符串"=w187) -> ("连接的字符串"=w186:string)  [unwired: 10 in]
      n121 = global write "全局 小时数据发送次数.vi" "小时数据发送次数"(w188) -> ()
      n122 = global write "全局1.vi" "枚举"(w188) -> ()
      n123 = global write "起始时间.vi" "结束时间"(w186) -> ()
      n124 = global write "起始时间.vi" "起始时间"(w184) -> ()
      n125 = flat-sequence {
        tunnel: [T1."发送数据" ("元素")] -> w182
        frame #0 {
          w193 = "提取集成干预" ("新元素/子数组")
          n126 = call "从数据库获取数据通用可配置(子VI).vi"("table输入"=w193, "列队名（唯一）"=w193) -> ()  [unwired: 8 in, 2 out]
        }
        frame #1 {
          n127 = call "数据处理整合 (子VI).vi"("枚举"=enum16{"实时数据排序", "小时数据排序"}."实时数据排序") -> ("已排序的数组"=w197:string[])  [unwired: 10 in]
          n128 = Array Size(array=w197) -> (size(s)=w196:i32)
          n129 = local write "table"("提取集成干预" ("新元素/子数组")) -> ()
          n130 = global write "全局 数据数组大小.vi" "数据数组大小"(w196) -> ()
        }
        frame #2 {
        }
      }
    }
    frame "3015" {
      n131 = flat-sequence {
        tunnel: [T1."发送数据" ("元素")] -> w199
        frame #0 {
          # "发命令给中控"
          # "发回给平台"
          # "3015、手动远程留样"
          n132 = local write "table"("超标留样返回" ("新元素/子数组")) -> ()
          n133 = Insert Into Array(array=u16[] [] ("holding register values"), index=0 ("索引"), new element=u16 1 ("新元素/子数组")) -> (w204:u16[])
          n134 = call "Modbus Master.vi"("Unit ID"=u8 1, "读取写入选择"="写入", "holding register values"=w204, "starting address"=u16 10) -> ()  [unwired: 6 in, 2 out]
        }
        frame #1 {
        }
      }
    }
    frame "3020" {
      n135 = flat-sequence {
        tunnel: [w223] -> w216
        tunnel: [w224] -> w215
        tunnel: [w222] -> w214
        tunnel: [w220] -> w213
        tunnel: w212 -> [w219]
        tunnel: [w219] -> w210
        tunnel: w216 -> [w272]
        tunnel: w215 -> [w271]
        tunnel: w214 -> [w270]
        tunnel: w213 -> [w269]
        tunnel: [w268] -> w211
        tunnel: w210 -> [w268]
        tunnel: [T1."发送数据" ("元素")] -> w217
        tunnel: w211 -> [w320]
        frame #0 {
          w242 = 0 ("数值")
          # "3020、提取日志、报警，仪器参数"
          n136 = Search/Split String(string=w219, search string/char (-)="BeginTime=" ("搜索字符串")) -> (match + rest of string=w241:string)  [unwired: 1 in, 2 out]
          n137 = case shown="\"\"" w241 {
            tunnel: ["1904/01/01 00:00:00" w265] -> w244
            tunnel: w241 -> [_ w259]
            tunnel: [w252 w260] -> w240
            frame "" {
              # "时间"
              n138 = Get Date/Time In Seconds() -> (seconds since 1Jan1904=w253:timestamp)
              n139 = Format Date/Time String(time format string (%c)="%Y%m%d%H%M%S%3u" ("时间格式字符串(%c)"), seconds (now)=w253) -> (date/time string=w257:string)  [unwired: 1 in]
              n140 = Search and Replace String(input string=w257, search string="." ("搜索字符串")) -> (result string=w256:string)  [unwired: 6 in, 3 out]
              n141 = call "格式时间字符串.vi"("字符串"=w256) -> ("连接的字符串"=w252:string)  [unwired: 10 in]
            }
            frame "真", Default {
              # "格式时间"
              n142 = String Subset(string=w259, offset (0)=33 ("偏移量(0)"), length (rest)=14 ("长度（剩余）")) -> (substring=w263:string)
              n143 = String Subset(string=w259, offset (0)=10 ("偏移量(0)"), length (rest)=14 ("长度（剩余）")) -> (substring=w264:string)
              n144 = call "格式时间字符串.vi"("字符串"=w263) -> ("连接的字符串"=w260:string)  [unwired: 10 in]
              n145 = call "格式时间字符串.vi"("字符串"=w264) -> ("连接的字符串"=w265:string)  [unwired: 10 in]
            }
          }
          n146 = call "日志报警参数选择 (子VI).vi"("String输入"=w219) -> ("输出簇"=w227:T3)  [unwired: 9 in, 1 out]
          n147 = Unbundle By Name(w227) -> ("高锰酸盐"=w234:string, "化学需氧量"=w235:string, "氨氮"=w236:string, "总磷"=w237:string, "总氮"=w238:string, "数采仪"=w239:string, "高锰酸盐"=w228:bool, "化学需氧量"=w229:bool, "氨氮"=w230:bool, "总磷"=w231:bool, "总氮"=w232:bool, "数采仪"=w233:bool)
          n148 = Build Array(w234, w235, w236, w237, w238, w239) -> (w222:string[])
          n149 = global write "全局 时间2.vi" "时间2"(w240) -> ()
          n150 = Build Array(w228, w229, w230, w231, w232, w233) -> (w221:bool[])
          n151 = global write "全局 水样时间.vi" "时间"(w244) -> ()
          n152 = Or Array Elements(Boolean array=w221) -> (logical OR=w220:bool)
          n153 = global write "全局 小时数据发送次数.vi" "小时数据发送次数"(w242) -> ()
          n154 = Obtain Queue(name (unnamed)="操作日志报警信息" ("名称（未命名）"), element data type=T2."CODMn") -> (queue out=w223:refnum<queue>, error out=w224:errorcluster)  [unwired: 3 in, 1 out]
          n155 = case shown="真" w220 {
            tunnel: w223 -> [_ w246]
            tunnel: w221 -> [_ w245]
            frame False {
            }
            frame True {
              n156 = for {
                tunnel: w245 -> [w248] mode=indexing
                tunnel: w246 -> [w247]
                i -> [w249]
                n157 = case shown="真" w248 {
                  tunnel: w249 -> [_ w251]
                  tunnel: w247 -> [_ w250]
                  frame False {
                  }
                  frame True {
                    n158 = call "提取日志报警参数入列队 (子VI).vi"("枚举"=w251, "queue in"=w250) -> ()  [unwired: 10 in]
                  }
                }
              }
            }
          }
          n159 = global write "全局1.vi" "枚举"(w242) -> ()
        }
        frame #1 {
          # "按需求提取COD、氨氮、总磷、总氮日志"
          # "按需求提取COD、氨氮、总磷、总氮日志"
          n160 = case shown="真" w269 {
            tunnel: w271 -> [_ w275]
            tunnel: w272 -> [_ w274]
            tunnel: w270 -> [_ w273]
            frame False {
            }
            frame True {
              n161 = while {
                shift-right: [w289] -> _
                shift-left: w274 -> [w290]
                tunnel: w275 -> [w288]
                tunnel: w273 -> [w283]
                stop <- w285 stop-if-true
                n162 = Dequeue Element(queue=w290, error in (no error)=w288) -> (queue out=w287:refnum<queue>, element=w282:T2)  [unwired: 1 in, 2 out]
                n163 = Index Array(array=w283) -> (element #1=w281:string, element #2=w280:string, element #3=w279:string, element #4=w278:string, element #5=w277:string, element #6=w276:string)  [unwired: 6 in]
                n164 = case shown="\"CODCr\"" w282 {
                  tunnel: w287 -> [w295 _ w304 w309 w313 w318]
                  tunnel: [w295 _ w304 w309 w313 w318] -> w289
                  tunnel: w281 -> [w292 _ _ _ _ _]
                  tunnel: w280 -> [_ w297 _ _ _ _]
                  tunnel: w279 -> [_ _ w301 _ _ _]
                  tunnel: w278 -> [_ _ _ w306 _ _]
                  tunnel: w277 -> [_ _ _ _ w311 _]
                  tunnel: w276 -> [_ _ _ _ _ w315]
                  frame "CODMn" {
                    w291 = string[][] [] ("氨氮")
                    n165 = call "数据表比对.vi"("仪器日志参数"="CODMn" ("元素"), "table输入"=w292) -> ("待发送数据"=w293:string[][])  [unwired: 7 in, 2 out]
                    n166 = global write "全局 所有参数.vi" "CODMn"(w293) -> ()
                    n167 = global write "全局 所有参数.vi" "总氮"(w291) -> ()
                    n168 = global write "全局 所有参数.vi" "CODCr"(w291) -> ()
                    n169 = global write "全局 所有参数.vi" "总磷"(w291) -> ()
                    n170 = global write "全局 所有参数.vi" "氨氮"(w291) -> ()
                  }
                  frame "CODCr" {
                    w296 = string[][] [] ("氨氮")
                    n171 = call "数据表比对.vi"("仪器日志参数"="CODCr" ("元素"), "table输入"=w297) -> ("待发送数据"=w298:string[][])  [unwired: 7 in, 2 out]
                    n172 = global write "全局 所有参数.vi" "CODCr"(w298) -> ()
                    n173 = global write "全局 所有参数.vi" "CODMn"(w296) -> ()
                    n174 = global write "全局 所有参数.vi" "总氮"(w296) -> ()
                    n175 = global write "全局 所有参数.vi" "总磷"(w296) -> ()
                    n176 = global write "全局 所有参数.vi" "氨氮"(w296) -> ()
                  }
                  frame "氨氮" {
                    w300 = string[][] [] ("氨氮")
                    n177 = call "数据表比对.vi"("仪器日志参数"="氨氮" ("元素"), "table输入"=w301) -> ("待发送数据"=w302:string[][])  [unwired: 7 in, 2 out]
                    n178 = global write "全局 所有参数.vi" "氨氮"(w302) -> ()
                    n179 = global write "全局 所有参数.vi" "CODMn"(w300) -> ()
                    n180 = global write "全局 所有参数.vi" "总氮"(w300) -> ()
                    n181 = global write "全局 所有参数.vi" "CODCr"(w300) -> ()
                    n182 = global write "全局 所有参数.vi" "总磷"(w300) -> ()
                  }
                  frame "总磷" {
                    w305 = string[][] [] ("氨氮")
                    n183 = call "数据表比对.vi"("仪器日志参数"="总磷" ("元素"), "table输入"=w306) -> ("待发送数据"=w307:string[][])  [unwired: 7 in, 2 out]
                    n184 = global write "全局 所有参数.vi" "总磷"(w307) -> ()
                    n185 = global write "全局 所有参数.vi" "CODMn"(w305) -> ()
                    n186 = global write "全局 所有参数.vi" "总氮"(w305) -> ()
                    n187 = global write "全局 所有参数.vi" "CODCr"(w305) -> ()
                    n188 = global write "全局 所有参数.vi" "氨氮"(w305) -> ()
                  }
                  frame "总氮" {
                    w310 = string[][] [] ("氨氮")
                    n189 = call "数据表比对.vi"("仪器日志参数"="总氮" ("元素"), "table输入"=w311) -> ("待发送数据"=w312:string[][])  [unwired: 7 in, 2 out]
                    n190 = global write "全局 所有参数.vi" "总氮"(w312) -> ()
                    n191 = global write "全局 所有参数.vi" "CODMn"(w310) -> ()
                    n192 = global write "全局 所有参数.vi" "氨氮"(w310) -> ()
                    n193 = global write "全局 所有参数.vi" "CODCr"(w310) -> ()
                    n194 = global write "全局 所有参数.vi" "总磷"(w310) -> ()
                  }
                  frame "数采仪" {
                    n195 = call "数据表比对.vi"("仪器日志参数"="系统" ("元素"), "table输入"=w315) -> ("待发送数据"=w316:string[][])  [unwired: 7 in, 2 out]
                    n196 = global write "全局 所有参数.vi" "DO"(w316) -> ()
                  }
                }
                n197 = Get Queue Status(queue=w287) -> (# elements in queue=w286:i32)  [unwired: 2 in, 7 out]
                n198 = Wait (ms)(milliseconds to wait=u32 300 ("等待时间（毫秒）")) -> ()  [unwired: 1 out]
                n199 = Equal To 0?(x=w286) -> (x = 0?=w285:bool)
              }
            }
          }
        }
        frame #2 {
          n200 = Search/Split String(string=w320, search string/char (-)="InfoId=" ("搜索字符串/字符(-)")) -> (match + rest of string=w326:string)  [unwired: 1 in, 2 out]
          n201 = String Subset(string=w326, offset (0)=7 ("偏移量(0)"), length (rest)=6 ("长度（剩余）")) -> (substring=w322:string)
          n202 = case shown="\"i13001\", \"i13002\", \"i13003\", \"i13004\", \"i13005\", \"i13006\", \"i13007\", \"i13008\", \"i13009\", \"i13010\", \"i13011\", \"i13012\", \"i13013\"" w322 {
            selector: w322 -> [_ w332 _]
            tunnel: ["操作日志" ("名称（未命名）") "提取仪器参数" ("名称（未命名）") "报警信息" ("名称（未命名）")] -> w319
            tunnel: [w328 1 ("数据数组大小") w335] -> w321
            frame "i11001", "i21001" {
              # "数据处理整合"
              # "i11001日志"
              n203 = call "数据处理整合 (子VI).vi"("枚举"=enum16{"实时数据排序", "小时数据排序"}."实时数据排序") -> ("已排序的数组"=w329:string[])  [unwired: 10 in]
              n204 = Array Size(array=w329) -> (size(s)=w328:i32)
            }
            frame "i13001", "i13002", "i13003", "i13004", "i13005", "i13006", "i13007", "i13008", "i13009", "i13010", "i13011", "i13012", "i13013" {
              n205 = global write "全局 提取仪器参数.vi" "参数编码"(w332) -> ()
              n206 = call "数据处理直接插入整合 (子VI).vi"() -> ()  [unwired: 12 in]
            }
            frame "i12001", Default {
              # "数据处理整合"
              # "i12001状态"
              n207 = call "数据处理整合 (子VI).vi"("枚举"=enum16{"实时数据排序", "小时数据排序"}."实时数据排序") -> ("已排序的数组"=w336:string[])  [unwired: 10 in]
              n208 = Array Size(array=w336) -> (size(s)=w335:i32)
            }
          }
          n209 = global write "全局 数据数组大小.vi" "数据数组大小"(w321) -> ()
          n210 = local write "table"(w319) -> ()
        }
      }
    }
    frame "3021" {
      # "设置仪表参数"
      n211 = local write "table"("反控命令" ("新元素/子数组")) -> ()
    }
    frame "3040" {
      # "提取现场系统信息（3040）"
      n212 = flat-sequence {
        tunnel: [T1."发送数据" ("元素")] -> w342
        frame #0 {
          n213 = local write "table"("提取现场系统信息" ("新元素/子数组")) -> ()
        }
        frame #1 {
        }
      }
    }
    frame "3041" {
      # "提取现场经纬度及环境信息（3041）"
      n214 = flat-sequence {
        tunnel: [T1."发送数据" ("元素")] -> w346
        frame #0 {
          n215 = call "获取环境参数 (子VI).vi"() -> ()  [unwired: 12 in]
          n216 = local write "table"("提取经纬度环境信息" ("新元素/子数组")) -> ()
        }
        frame #1 {
        }
      }
    }
    frame "3042" {
      # "发命令给中控"
      # "反控指令"
      # "0维护，1常规，2应急，3质控"
      # "反控指令\n切换运行模式"
      n217 = local write "table"("反控命令" ("新元素/子数组")) -> ()
      n218 = Search/Split String(string=w351, search string/char (-)="RunMode" ("搜索字符串/字符(-)")) -> (match + rest of string=w364:string)  [unwired: 1 in, 2 out]
      n219 = String Subset(string=w364, offset (0)=8 ("偏移量(0)"), length (rest)=1 ("长度（剩余）")) -> (substring=w361:string)
      n220 = case shown="\"2\"" w361 {
        tunnel: [u16 0 ("新元素/子数组") u16 1 ("新元素/子数组") u16 2 ("新元素/子数组") u16 3 ("新元素/子数组")] -> w356
        frame "0", Default {
        }
        frame "1" {
        }
        frame "2" {
        }
        frame "3" {
        }
      }
      n221 = Insert Into Array(array=u16[] [] ("holding register values"), index=0 ("索引"), new element=w356) -> (w357:u16[])
      n222 = call "Modbus Master.vi"("Unit ID"=u8 1, "读取写入选择"="写入", "holding register values"=w357, "starting address"=u16 0) -> ()  [unwired: 6 in, 2 out]
    }
    frame "3043" {
      # "远程重启数采仪"
      n223 = local write "table"("反控命令" ("新元素/子数组")) -> ()
    }
    frame "3044" {
      # "发回给平台"
      # "反控指令"
      # "3042~3086"
      # "反控指令\n单次测量"
      # "3044"
      n224 = local write "table"("反控命令" ("新元素/子数组")) -> ()
      n225 = flat-sequence {
        frame #0 {
          # "发命令给中控"
          n226 = call "Modbus Master.vi"("Unit ID"=u8 1, "读取写入选择"="写入", "holding register values"=u16[] [1], "starting address"=u16 2) -> ()  [unwired: 6 in, 2 out]
        }
        frame #1 {
          n227 = Wait (ms)(milliseconds to wait=u32 500 ("等待时间（毫秒）")) -> ()  [unwired: 1 out]
        }
        frame #2 {
          n228 = call "Modbus Master.vi"("Unit ID"=u8 1, "读取写入选择"="写入", "holding register values"=u16[] [0], "starting address"=u16 2) -> ()  [unwired: 6 in, 2 out]
        }
      }
    }
    frame "3045", "3046" {
      # "发回给平台"
      # "反控指令"
      # "3042~3086"
      # "反控指令\n急停"
      # "3045"
      n229 = flat-sequence {
        frame #0 {
          # "发命令给中控"
          n230 = call "Modbus Master.vi"("Unit ID"=u8 1, "读取写入选择"="写入", "holding register values"=u16[] [1], "starting address"=u16 3) -> ()  [unwired: 6 in, 2 out]
        }
        frame #1 {
          n231 = Wait (ms)(milliseconds to wait=u32 500 ("等待时间（毫秒）")) -> ()  [unwired: 1 out]
        }
        frame #2 {
          n232 = call "Modbus Master.vi"("Unit ID"=u8 1, "读取写入选择"="写入", "holding register values"=u16[] [0], "starting address"=u16 3) -> ()  [unwired: 6 in, 2 out]
        }
      }
      n233 = local write "table"("反控命令" ("新元素/子数组")) -> ()
    }
    frame "3056" {
      # "发命令给中控"
      # "设置测量时间间隔"
      # "发回给平台"
      n234 = local write "table"("反控命令" ("新元素/子数组")) -> ()
      n235 = Search/Split String(string=w398, search string/char (-)="RunInterval" ("搜索字符串/字符(-)")) -> (match + rest of string=w405:string)  [unwired: 1 in, 2 out]
      n236 = Decimal String To Number(string=w405, offset=12 ("偏移量(0)")) -> (number=w401:i32)  [unwired: 1 in, 1 out]
      n237 = Insert Into Array(array=u16[] [] ("holding register values"), index=0 ("索引"), new element=w401) -> (w400:u16[])
      n238 = call "Modbus Master.vi"("Unit ID"=u8 1, "读取写入选择"="写入", "holding register values"=w400, "starting address"=u16 14) -> ()  [unwired: 6 in, 2 out]
    }
    frame "3080", "3081", "3082", "3083", "3084", "3085", "3086" {
      # "30 启动标液核查  1CODmn  2 氨氮  3总磷  4总氮  5CODCr\n31 加标回收\n32 平行样测试\n33 零点核查\n34 跨度核查\n35 校零\n36 校标"
      # "发回给平台"
      n239 = flat-sequence {
        tunnel: w415 -> [w421]
        tunnel: [w419] -> w414
        tunnel: w412 -> [w418]
        tunnel: w414 -> [w446]
        tunnel: [w446] -> w413
        tunnel: w413 -> [w449]
        frame #0 {
          # "1CODmn  2 氨氮  3总磷  4总氮  5CODCr"
          # "启动单台仪器标液核查"
          # "发命令给中控"
          n240 = Search/Split String(string=w418, search string/char (-)="PolId" ("搜索字符串/字符(-)")) -> (match + rest of string=w426:string)  [unwired: 1 in, 2 out]
          n241 = String Subset(string=w426, offset (0)=6 ("偏移量(0)"), length (rest)=6 ("长度（剩余）")) -> (substring=w423:string)
          n242 = case shown="\"w01019\"" w423 {
            tunnel: [0 ("长度（剩余）") 1 ("长度（剩余）") 2 ("长度（剩余）") 3 ("长度（剩余）") 4 ("长度（剩余）") 5 ("长度（剩余）")] -> w422
            frame "", Default {
            }
            frame "w01019" {
            }
            frame "w21003" {
            }
            frame "w21011" {
            }
            frame "w21001" {
            }
            frame "w01018" {
            }
          }
          n243 = Insert Into Array(array=u16[] [] ("holding register values"), index=0 ("索引"), new element=w422) -> (w427:u16[])
          n244 = case shown="\"3086\"" w421 {
            tunnel: [u16 99 ("starting address") u16 30 ("starting address") u16 31 ("starting address") u16 32 ("starting address") u16 33 ("starting address") u16 34 ("starting address") u16 35 ("starting address") u16 36 ("starting address")] -> w419
            frame "", Default {
            }
            frame "3080" {
            }
            frame "3081" {
            }
            frame "3082" {
            }
            frame "3083" {
            }
            frame "3084" {
            }
            frame "3085" {
            }
            frame "3086" {
            }
          }
          n245 = call "Modbus Master.vi"("Unit ID"=u8 1, "读取写入选择"="写入", "holding register values"=w427, "starting address"=w419) -> ()  [unwired: 6 in, 2 out]
        }
        frame #1 {
          n246 = Wait (ms)(milliseconds to wait=u32 500 ("等待时间（毫秒）")) -> ()  [unwired: 1 out]
        }
        frame #2 {
          n247 = call "Modbus Master.vi"("Unit ID"=u8 1, "读取写入选择"="写入", "holding register values"=u16[] [0], "starting address"=w449) -> ()  [unwired: 6 in, 2 out]
        }
      }
      n248 = local write "table"("反控命令" ("新元素/子数组")) -> ()
    }
  }
  "元素" <- w3
  "队列输出" <- w2
